vi "FeuRougeVar.vi"() -> ()   [LabVIEW 2018]
panel:
  in  "4":dbl
  in  "3":dbl
  in  "2":dbl
  in  "1":dbl
  # "Durée des phases en secondes"
  # "Phase 1"
  # "Phase 2"
  # "Phase 3"
  # "Phase 4"
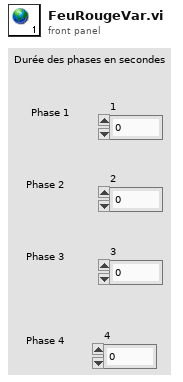
[diagram p1: front panel]
diagram:
